vi "Read Roles.vi"(8 "error in (no error)":errorcluster, 11 "SimpleBallPlacementAllyPlay in":refnum<class "SimpleBallPlacementAllyPlay.lvclass">) -> (0 "error out":errorcluster, 2 "Roles":T1, 3 "SimpleBallPlacementAllyPlay out":refnum<class "SimpleBallPlacementAllyPlay.lvclass">)   [LabVIEW 2021, in "SimpleBallPlacementAllyPlay.lvclass"]
uses:
  SimpleBallPlacementAllyPlay.lvclass
  RolesSimpleBallPlacementAllyPlay.ctl
  BallPlacementEnemyRole_class/BallPlacementEnemyRole.lvclass
  SimpleBallPlacementAllyRole_class/SimpleBallPlacementAllyRole.lvclass
  SimpleBallPlacementAllyPlay.lvclass/SimpleBallPlacementAllyPlay.ctl
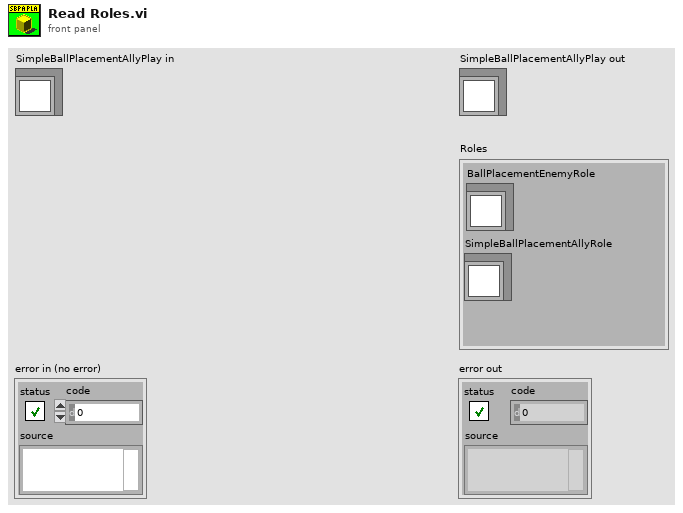
[diagram p1: front panel]
types:
  T1 = typedef "SimpleBallPlacementAllyPlay.lvclass/RolesSimpleBallPlacementAllyPlay.ctl" = cluster{"BallPlacementEnemyRole":refnum<class "BallPlacementEnemyRole.lvclass">, "SimpleBallPlacementAllyRole":refnum<class "SimpleBallPlacementAllyRole.lvclass">}
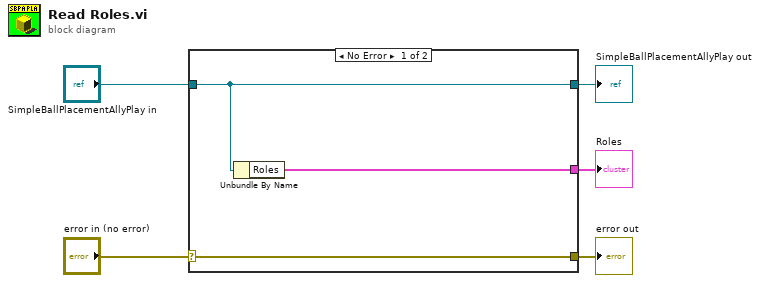
[diagram p0: block diagram]
diagram:
  n1 = case shown="No Error" "error in (no error)" {
    selector: "error in (no error)" -> [w8 w9]
    tunnel: [w8 w9] -> w4
    tunnel: [w7 w10] -> w2
    tunnel: "SimpleBallPlacementAllyPlay in" -> [w7 w10]
    tunnel: [w6 _] -> w1
    frame No Error {
      n2 = Unbundle By Name(w7) -> ("Roles"=w6:T1)
    }
    frame Error {
    }
  }
  "error out" <- w4
  "SimpleBallPlacementAllyPlay out" <- w2
  "Roles" <- w1
